vi "File to Element.vi"(10 "Element In":T1, 11 "Data In":string[](array[string])) -> (2 "Data Out":string[](array[string]), 3 "Element Out":T1)   [LabVIEW 2020]
uses:
  Global/Data Global/SDQ Data Type.ctl
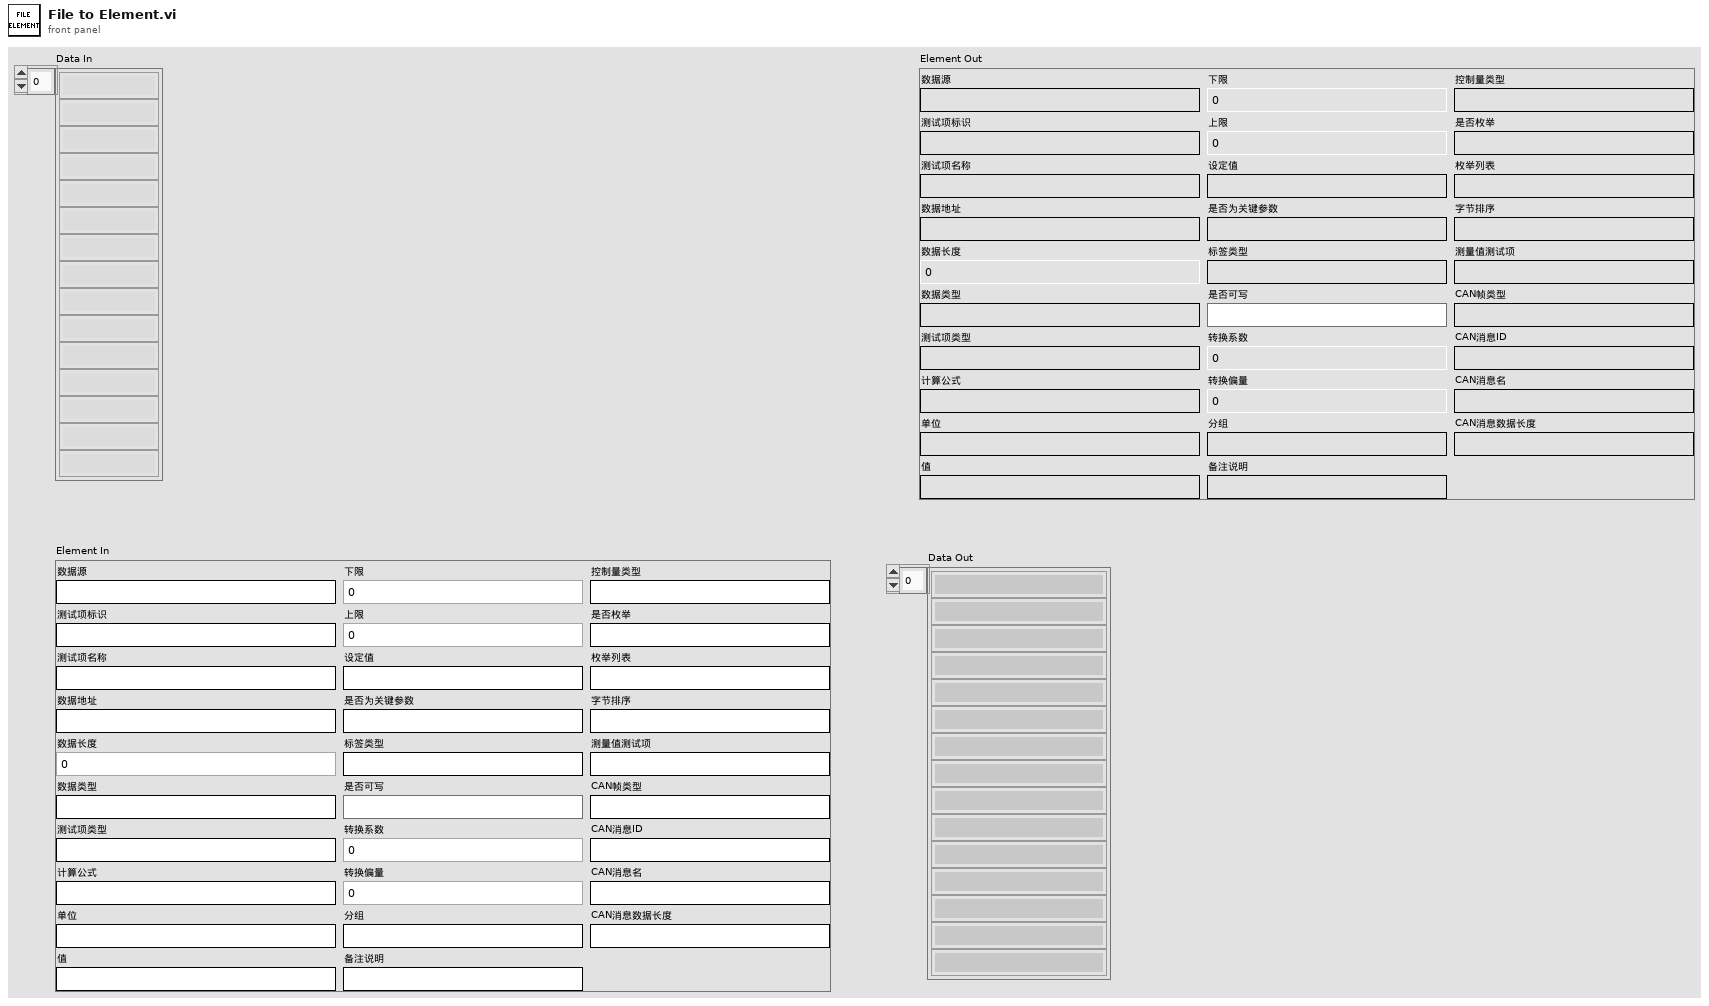
[diagram p1: front panel]
types:
  T1 = typedef "SDQ Data Type.ctl" = cluster{"CAN Length":string, "CAN Name":string, "CAN ID":string, "CAN Type":string, "Test Item":string, "Byte Order":string, "Instruction":string, "Control Type":string, "Group":string, "Offset":dbl, "Coefficient":dbl, "Write Enable":bool, "Lable Type":string, "Key?":string, "Set Value":string, "Upper":dbl, "Lower":dbl, "Unit":string, "Formula":string, "Test Item Type":string, "Length":i32, "Address":string, "Name":string, "Identifier":string, "Data Type":string, "Enumerate?":string, "Enumerate List":string, "Data":string, "Source":string}
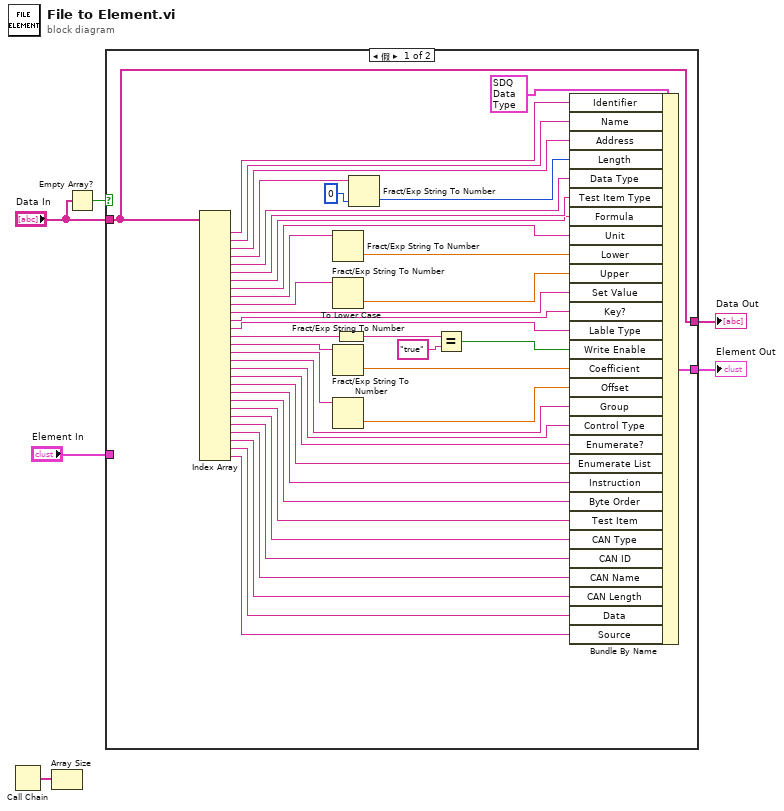
[diagram p0: block diagram]
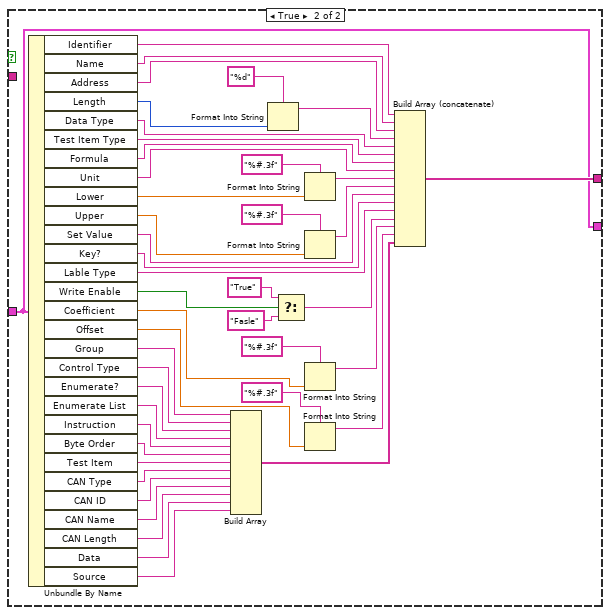
[diagram p2: hidden frame]
diagram:
  n1 = Call Chain() -> (call chain=w1:string[])
  n2 = Array Size(array=w1) -> ()  [unwired: 1 out]
  n3 = Empty Array?(array="Data In") -> (empty?=w4:bool)
  n4 = case shown="假" w4 {
    tunnel: [w47 w49] -> w6
    tunnel: "Data In" -> [w8 _]
    tunnel: "Element In" -> [_ w49]
    tunnel: [w8 w91] -> w2
    frame False {
      n5 = Index Array(array=w8) -> (element #1=w44:string, element #2=w25:string, element #3=w26:string, element #4=w27:string, element #5=w24:string, element #6=w23:string, element #7=w13:string, element #8=w14:string, element #9=w37:string, element #10=w40:string, element #11=w45:string, element #12=w15:string, element #13=w16:string, element #14=w41:string, element #15=w17:string, element #16=w20:string, element #17=w21:string, element #18=w22:string, element #19=w28:string, element #20=w29:string, element #21=w30:string, element #22=w31:string, element #23=w32:string, element #24=w33:string, element #25=w34:string, element #26=w35:string, element #27=w36:string, element #28=w10:string, element #29=w9:string)  [unwired: 29 in]
      n6 = Fract/Exp String To Number(string=w37) -> (number=w38:dbl)  [unwired: 3 in, 1 out]
      n7 = Fract/Exp String To Number(string=w40) -> (number=w39:dbl)  [unwired: 3 in, 1 out]
      n8 = Fract/Exp String To Number(string=w17) -> (number=w18:dbl)  [unwired: 3 in, 1 out]
      n9 = Fract/Exp String To Number(string=w20) -> (number=w19:dbl)  [unwired: 3 in, 1 out]
      n10 = To Lower Case(string=w41) -> (all lower case string=w7:string)
      n11 = Fract/Exp String To Number(string=w27, default (0 dbl)=0 ("数字后偏移量")) -> (number=w12:i32)  [unwired: 2 in, 1 out]
      n12 = Equal?(x=w7, y="true") -> (x = y?=w43:bool)
      n13 = Bundle By Name(cluster=T1 {"CAN Length"="", "CAN Name"="", "CAN ID"="", "CAN Type"="", "Test Item"="", "Byte Order"="", "Instruction"="", "Control Type"="", "Group"="", "Offset"=0.0, "Coefficient"=0.0, "Write Enable"=FALSE, "Lable Type"="", "Key?"="", "Set Value"="", "Upper"=0.0, "Lower"=0.0, "Unit"="", "Formula"="", "Test Item Type"="", "Length"=0, "Address"="", "Name"="", "Identifier"="", "Data Type"="", "Enumerate?"="", "Enumerate List"="", "Data"="", "Source"=""}, "Identifier"=w44, "Name"=w25, "Address"=w26, "Length"=w12, "Data Type"=w24, "Test Item Type"=w23, "Formula"=w13, "Unit"=w14, "Lower"=w38, "Upper"=w39, "Set Value"=w45, "Key?"=w15, "Lable Type"=w16, "Write Enable"=w43, "Coefficient"=w18, "Offset"=w19, "Group"=w21, "Control Type"=w22, "Enumerate?"=w28, "Enumerate List"=w29, "Instruction"=w30, "Byte Order"=w31, "Test Item"=w32, "CAN Type"=w33, "CAN ID"=w34, "CAN Name"=w35, "CAN Length"=w36, "Data"=w10, "Source"=w9) -> (w47:T1)
    }
    frame True {
      n14 = Unbundle By Name(w49) -> ("Identifier"=w92:string, "Name"=w90:string, "Address"=w89:string, "Length"=w87:i32, "Data Type"=w85:string, "Test Item Type"=w48:string, "Formula"=w84:string, "Unit"=w83:string, "Lower"=w81:dbl, "Upper"=w78:dbl, "Set Value"=w76:string, "Key?"=w75:string, "Lable Type"=w74:string, "Write Enable"=w73:bool, "Coefficient"=w68:dbl, "Offset"=w65:dbl, "Group"=w63:string, "Control Type"=w62:string, "Enumerate?"=w61:string, "Enumerate List"=w60:string, "Instruction"=w59:string, "Byte Order"=w58:string, "Test Item"=w57:string, "CAN Type"=w56:string, "CAN ID"=w55:string, "CAN Name"=w54:string, "CAN Length"=w53:string, "Data"=w52:string, "Source"=w51:string)
      n15 = Build Array(w63, w62, w61, w60, w59, w58, w57, w56, w55, w54, w53, w52, w51) -> (w50:string[])
      n16 = Format Into String(format string="%d" ("格式字符串"), w87) -> (resulting string=w86:string)  [unwired: 2 in, 1 out]
      n17 = Select(t="True", s=w73, f="Fasle") -> (s? t:f=w70:string)
      n18 = Format Into String(format string="%#.3f" ("格式字符串"), w81) -> (resulting string=w80:string)  [unwired: 2 in, 1 out]
      n19 = Format Into String(format string="%#.3f" ("格式字符串"), w78) -> (resulting string=w77:string)  [unwired: 2 in, 1 out]
      n20 = Format Into String(format string="%#.3f" ("格式字符串"), w68) -> (resulting string=w67:string)  [unwired: 2 in, 1 out]
      n21 = Format Into String(format string="%#.3f" ("格式字符串"), w65) -> (resulting string=w64:string)  [unwired: 2 in, 1 out]
      n22 = Build Array (concatenate)(w92, w90, w89, w86, w85, w48, w84, w83, w80, w77, w76, w75, w74, w70, w67, w64, w50) -> (w91:string[])
    }
  }
  "Element Out" <- w6
  "Data Out" <- w2
